vi "Load Fuzzy Controller.vi"(5 "File Path":path, 7 "Open-Dialog":string="Open...") -> (0 "Controller out":T1={"Parameters"={"antecedance"=[{"ling.var."="Fuzzy-IN II", "x-min"=-10.0, "x-max"=10.0, "setarray"=[{"linguistic term"="NB", "color"=16711680, "points"=[-1.0, -1.0, -0.09999999999999998, -0.050000000000000044]}, {"linguistic term"="NS", "color"=3342438, "points"=[-0.09999999999999998, -0.050000000000000044, -0.050000000000000044, 0.0]}, {"linguistic term"="ZE", "color"=16724991, "points"=[-0.050000000000000044, 0.0, 0.0, 0.050000000000000044]}, {"linguistic term"="PS", "color"=255, "points"=[0.0, 0.050000000000000044, 0.050000000000000044, 0.10000000000000009]}, {"linguistic term"="PB", "color"=26214, "points"=[0.050000000000000044, 0.10000000000000009, 1.0, 1.0]}]}], "consequence"=[{"ling.var."="Fuzzy-OUT II", "x-min"=-10.0, "x-max"=10.0, "setarray"=[{"linguistic term"="NV", "color"=16711680, "points"=[-1.0, -1.0, -1.0, -1.0]}, {"linguistic term"="NED", "color"=3342438, "points"=[-0.5, -0.5, -0.5, -0.5]}, {"linguistic term"="NU", "color"=16724991, "points"=[0.0, 0.0, 0.0, 0.0]}, {"linguistic term"="PED", "color"=255, "points"=[0.5, 0.5, 0.5, 0.5]}, {"linguistic term"="PV", "color"=26214, "points"=[1.0, 1.0, 1.0, 1.0]}]}], "conclusions"=[0, 1, 2, 3, 4], "degree-of-support"=[1.0, 1.0, 1.0, 1.0, 1.0], "defu"=[{"inference"=0, "defumethod"=2, "modification"=TRUE, "precision"=0, "no consequence"=0, "defaultvalue"=0.0}]}, "Description"={"Info"={"Path"=path "/Mac IIsi/Work IIsi/Carsten&Stefan/Controller/Behaelter_P2.fc", "Controller Name"="Behaelter_P2.fc", "Date"="02.07.1996", "Time"="10:49 Uhr"}, "Author"="", "Description"=""}} {"Parameters"."defu"."defaultvalue" format="%.2f"; "Parameters"."degree-of-support" step=0.009999999776482582 format="%.2f"; "Parameters"."consequence"."x-min" step=0.009999999776482582 format="%.2f"; "Parameters"."consequence"."x-max" step=0.009999999776482582 format="%.2f"; "Parameters"."consequence"."setarray"."points" step=0.009999999776482582 format="%.2f"; "Parameters"."antecedance"."x-min" step=0.009999999776482582 format="%.2f"; "Parameters"."antecedance"."x-max" step=0.009999999776482582 format="%.2f"; "Parameters"."antecedance"."setarray"."points" step=0.009999999776482582 format="%.2f"}, 1 "cancel":bool, 2 "error out":errorcluster, 3 "anteced. data range minimums":dbl[](array[numeric]) format="%.2f", 4 "anteced. data range maximums":dbl[](array[numeric]) format="%.2f", 6 "input name 1":string, 8 "min 1":dbl format="%.2f", 10 "input name 2":string, 11 "min 4":dbl format="%.2f", 12 "input name 4":string, 13 "min 3":dbl format="%.2f", 14 "input name 3":string, 15 "min 2":dbl format="%.2f")   [LabVIEW 2020, in "NI_fuzzy logic.lvlib"]
doc: "This VI loads all controller parameters and information. Use this VI together with Fuzzy Controller VI to implement a fuzzy controller designed with the Fuzzy Logic Controller Design project manager. The data file uses the .fc file extension."
uses:
  <vilib>/addons/control/fuzzy/NI_fuzzy logic.lvlib
  <vilib>/addons/control/fuzzy/fuzzy logic.llb/Fuzzy Datatype.ctl
panel:
  in  "error in (not an error)":errorcluster
  in  "Controller data":T2={"Parameters"={"antecedance"=[{"ling.var."="in1", "x-min"=-1.0, "x-max"=1.0, "setarray"=[{"linguistic term"="NE1", "color"=16711680, "points"=[-1.0, -1.0, -1.0, -2.2351741790771484e-05]}, {"linguistic term"="ZE1", "color"=255, "points"=[-1.0, 0.0, 0.0, 1.0]}, {"linguistic term"="PO1", "color"=26214, "points"=[0.0, 1.0, 1.0, 1.0]}]}, {"ling.var."="in2", "x-min"=-1.0, "x-max"=1.0, "setarray"=[{"linguistic term"="NE2", "color"=16711680, "points"=[-1.0, -1.0, -1.0, 0.0]}, {"linguistic term"="ZE2", "color"=255, "points"=[-1.0, 0.0, 0.0, 1.0]}, {"linguistic term"="PO2", "color"=26214, "points"=[0.0, 1.0, 1.0, 1.0]}]}], "consequence"=[{"ling.var."="out", "x-min"=-1.0, "x-max"=1.0, "setarray"=[{"linguistic term"="NEo", "color"=16711680, "points"=[-1.0, -1.0, -1.0, 0.0]}, {"linguistic term"="ZEo", "color"=255, "points"=[-1.0, 0.0, 0.0, 1.0]}, {"linguistic term"="POo", "color"=26214, "points"=[0.0, 1.0, 1.0, 1.0]}]}], "conclusions"=[3, 3, 3, 3, 3, 3, 3], "degree-of-support"=[1.0, 1.0, 1.0, 1.0, 1.0, 1.0, 1.0], "defu"=[{"inference"=0, "defumethod"=0, "modification"=TRUE, "precision"=0, "no consequence"=0, "defaultvalue"=0.0}]}, "Description"={"Info"={"Path"=path "/HD 1000/Desktop Folder/fuzzylab today/loadsave.vi", "Controller Name"="", "Date"="", "Time"=""}, "Author"="", "Text"=""}} {"Parameters"."defu"."defaultvalue" format="%.2f"; "Parameters"."degree-of-support" step=0.009999999776482582 format="%.2f"; "Parameters"."consequence"."x-min" step=0.009999999776482582 format="%.2f"; "Parameters"."consequence"."x-max" step=0.009999999776482582 format="%.2f"; "Parameters"."consequence"."setarray"."points" step=0.009999999776482582 format="%.2f"; "Parameters"."antecedance"."x-min" step=0.009999999776482582 format="%.2f"; "Parameters"."antecedance"."x-max" step=0.009999999776482582 format="%.2f"; "Parameters"."antecedance"."setarray"."points" step=0.009999999776482582 format="%.2f"}
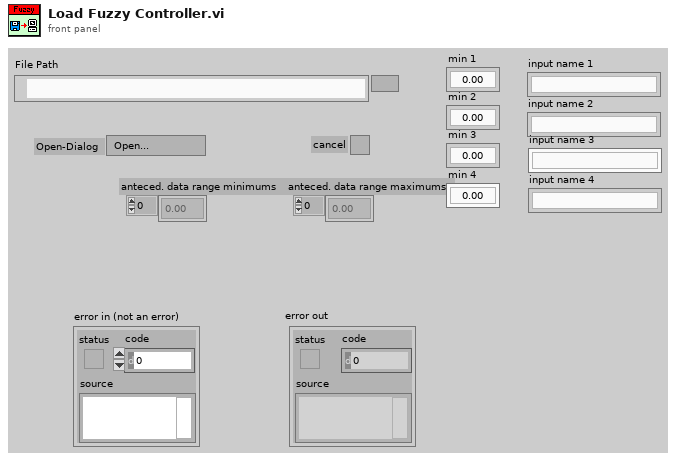
[diagram p1: front panel]
types:
  T1 = typedef "NI_fuzzy logic.lvlib/Fuzzy Datatype.ctl" = cluster{"Parameters":cluster{"antecedance":cluster{"ling.var.":string, "x-min":dbl, "x-max":dbl, "setarray":cluster{"linguistic term":string, "color":u32, "points":dbl[]}[]}[], "consequence":cluster{"ling.var.":string, "x-min":dbl, "x-max":dbl, "setarray":cluster{"linguistic term":string, "color":u32, "points":dbl[]}[]}[], "conclusions":u16[], "degree-of-support":dbl[], "defu":cluster{"inference":u16, "defumethod":u16, "modification":bool, "precision":u16, "no consequence":u16, "defaultvalue":dbl}[]}, "Description":cluster{"Info":cluster{"Path":path, "Controller Name":string, "Date":string, "Time":string}, "Author":string, "Description":string}}
  T2 = cluster{"Parameters":cluster{"antecedance":cluster{"ling.var.":string, "x-min":dbl, "x-max":dbl, "setarray":cluster{"linguistic term":string, "color":u32, "points":dbl[]}[]}[], "consequence":cluster{"ling.var.":string, "x-min":dbl, "x-max":dbl, "setarray":cluster{"linguistic term":string, "color":u32, "points":dbl[]}[]}[], "conclusions":u16[], "degree-of-support":dbl[], "defu":cluster{"inference":u16, "defumethod":u16, "modification":bool, "precision":u16, "no consequence":u16, "defaultvalue":dbl}[]}, "Description":cluster{"Info":cluster{"Path":path, "Controller Name":string, "Date":string, "Time":string}, "Author":string, "Text":string}}
  T3 = enum16{"open", "replace", "create", "open or create", "replace or create", "replace or create with confirmation"}
  T4 = cluster{"ling.var.":string, "x-min":dbl, "x-max":dbl, "setarray":cluster{"linguistic term":string, "color":u32, "points":dbl[]}[]}[]
  T5 = cluster{"inference":u16, "defumethod":u16, "modification":bool, "precision":u16, "no consequence":u16, "defaultvalue":dbl}[]
  T6 = cluster{"inference":u16, "defumethod":u16, "modification":bool, "precision":u16, "no consequence":u16, "defaultvalue":dbl}
  T7 = cluster{"linguistic term":string, "color":u32, "points":dbl[]}[]
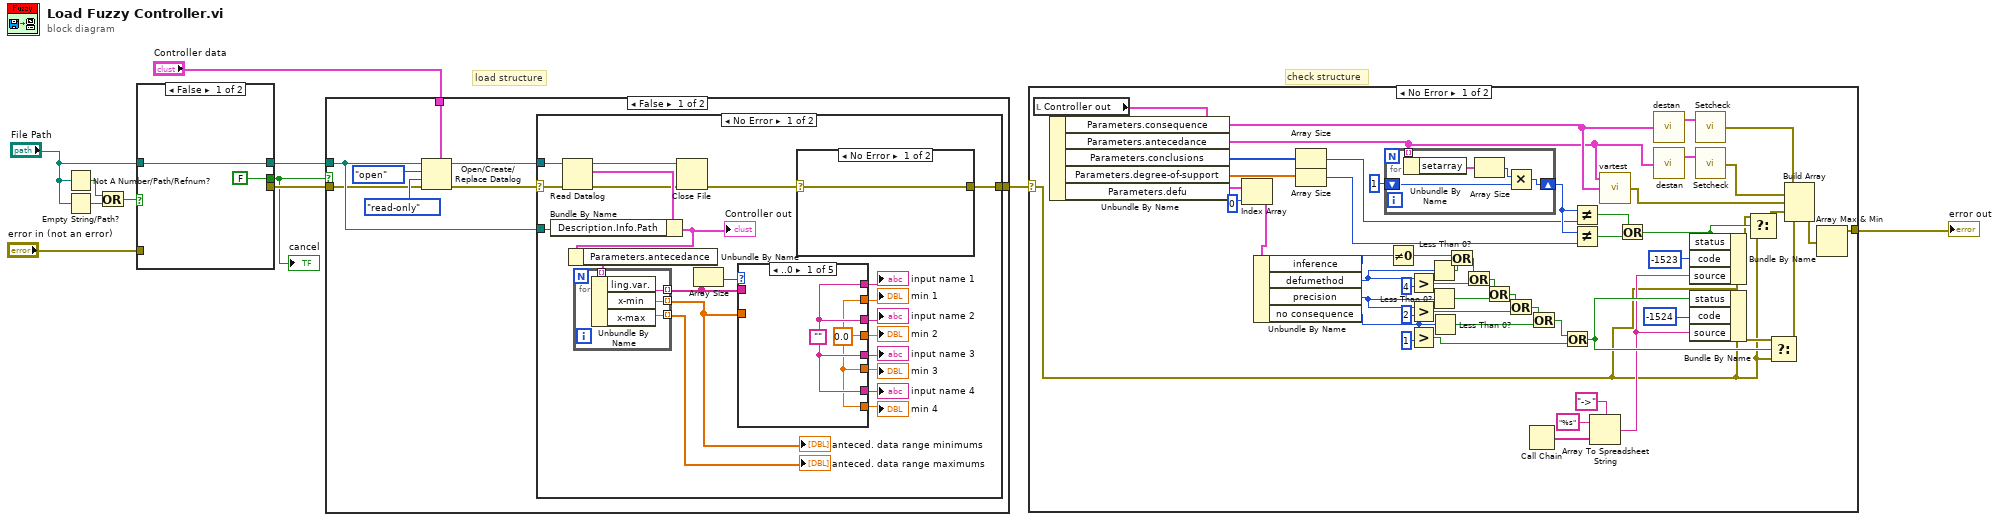
[diagram p0: block diagram]
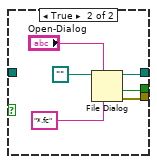
[diagram p2: hidden frame]
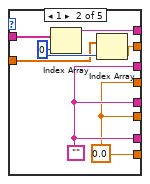
[diagram p4: hidden frame]
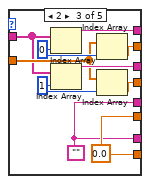
[diagram p5: hidden frame]
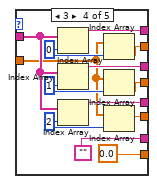
[diagram p6: hidden frame]
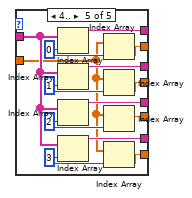
[diagram p7: hidden frame]
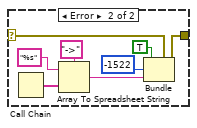
[diagram p8: hidden frame]
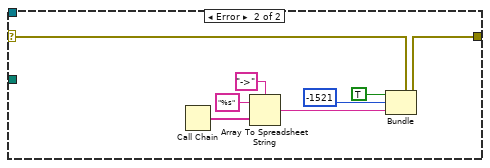
[diagram p9: hidden frame]
diagram:
  # "check structure"
  # "load structure"
  n1 = Not A Number/Path/Refnum?(number/path/refnum="File Path") -> (NaN/Path/Refnum?=w6:bool)
  n2 = Empty String/Path?(string/path="File Path") -> (empty?=w5:bool)
  n3 = Or(x=w6, y=w5) -> (x .or. y?=w3:bool)
  n4 = case shown="False" w3 {
    tunnel: [w13 w17] -> w9
    tunnel: [_ w19] -> w8
    tunnel: [FALSE ("cancelled") w18] -> w7
    tunnel: "File Path" -> [w13 _]
    tunnel: "error in (not an error)" -> [_ _]
    frame False {
    }
    frame True {
      n5 = File Dialog(6:"*.fc", 7:"Open-Dialog", 11:path "") -> (0:w19:errorcluster, 1:w18:bool, 3:w17:path)  [unwired: 1 in, 4 out]
    }
  }
  "cancel" <- w7
  n6 = case shown="False" w7 {
    tunnel: w9 -> [w25 _]
    tunnel: [w26 _] -> w1
    tunnel: "Controller data" -> [w24 _]
    tunnel: w8 -> [w21 _]
    frame False {
      n7 = Open/Create/Replace Datalog(5:w24, 8:w21, 9:enum16{"read/write", "read-only", "write-only"}."read-only" ("access (0:read/write)"), 10:T3."open" ("operation (0:open)"), 11:w25) -> (0:w20:errorcluster, 3:w27:refnum<k1>)  [unwired: 2 out]
      n8 = case shown="No Error" w20 {
        selector: w20 -> [w29 w113]
        tunnel: w27 -> [w49 _]
        tunnel: [w28 w109] -> w26
        tunnel: w25 -> [w46 _]
        frame No Error {
          n9 = Read Datalog(4:w29, 7:w49) -> (0:w31:errorcluster, 2:w47:T2, 3:w48:refnum<k1>)  [unwired: 1 out]
          n10 = Bundle By Name(cluster=w47, "Description.Info.Path"=w46) -> (w45:T2)
          "Controller out" <- w45
          n11 = Unbundle By Name(w45) -> ("Parameters.antecedance"=w44:T4)
          n12 = for {
            tunnel: w44 -> [w99] mode=indexing
            tunnel: [w98] -> w42 mode=indexing
            tunnel: [w97] -> w37 mode=indexing
            tunnel: [w96] -> w36 mode=indexing
            n13 = Unbundle By Name(w99) -> ("ling.var."=w98:string, "x-min"=w97:dbl, "x-max"=w96:dbl)
          }
          "anteced. data range minimums" <- w37
          "anteced. data range maximums" <- w36
          n14 = Close File(refnum=w48, error in=w31) -> (error out=w30:errorcluster)  [unwired: 1 out]
          n15 = Array Size(array=w42) -> (size(s)=w43:i32)
          n16 = case shown="..0" w43 {
            tunnel: w42 -> [_ w54 w60 w77 w90]
            tunnel: [w51 w58 w68 w81 w95] -> w41
            tunnel: [w51 w53 w66 w79 w93] -> w40
            tunnel: [w51 w53 w59 w78 w92] -> w39
            tunnel: [w51 w53 w59 "" w91] -> w38
            tunnel: w37 -> [_ w55 w62 w71 w82]
            tunnel: [w50 w56 w64 w74 w86] -> w35
            tunnel: [w50 w52 w63 w73 w85] -> w34
            tunnel: [w50 w52 w61 w72 w84] -> w33
            tunnel: [w50 w52 w61 0.0 w83] -> w32
            frame ..0 {
              w50 = 0.0
              w51 = ""
            }
            frame 1 {
              w52 = 0.0
              w53 = ""
              w57 = 0
              n17 = Index Array(array=w54, index=w57) -> (element=w58:string)
              n18 = Index Array(array=w55, index=w57) -> (element=w56:dbl)
            }
            frame 2 {
              w61 = 0.0
              w59 = ""
              w65 = 1
              w67 = 0
              n19 = Index Array(array=w60, index=w67) -> (element=w68:string)
              n20 = Index Array(array=w60, index=w65) -> (element=w66:string)
              n21 = Index Array(array=w62, index=w67) -> (element=w64:dbl)
              n22 = Index Array(array=w62, index=w65) -> (element=w63:dbl)
            }
            frame 3 {
              w75 = 2
              w76 = 1
              w80 = 0
              n23 = Index Array(array=w77, index=w80) -> (element=w81:string)
              n24 = Index Array(array=w77, index=w76) -> (element=w79:string)
              n25 = Index Array(array=w77, index=w75) -> (element=w78:string)
              n26 = Index Array(array=w71, index=w80) -> (element=w74:dbl)
              n27 = Index Array(array=w71, index=w76) -> (element=w73:dbl)
              n28 = Index Array(array=w71, index=w75) -> (element=w72:dbl)
            }
            frame 4.. {
              w87 = 3
              w88 = 2
              w89 = 1
              w94 = 0
              n29 = Index Array(array=w90, index=w94) -> (element=w95:string)
              n30 = Index Array(array=w90, index=w89) -> (element=w93:string)
              n31 = Index Array(array=w90, index=w88) -> (element=w92:string)
              n32 = Index Array(array=w90, index=w87) -> (element=w91:string)
              n33 = Index Array(array=w82, index=w94) -> (element=w86:dbl)
              n34 = Index Array(array=w82, index=w89) -> (element=w85:dbl)
              n35 = Index Array(array=w82, index=w88) -> (element=w84:dbl)
              n36 = Index Array(array=w82, index=w87) -> (element=w83:dbl)
            }
          }
          "input name 4" <- w38
          "input name 3" <- w39
          "input name 2" <- w40
          "input name 1" <- w41
          "min 4" <- w32
          "min 3" <- w33
          "min 2" <- w34
          "min 1" <- w35
          n37 = case shown="No Error" w30 {
            selector: w30 -> [w100 w103]
            tunnel: [w100 w101] -> w28
            frame No Error {
            }
            frame Error {
              n38 = Call Chain() -> (call chain=w106:string[])
              n39 = Array To Spreadsheet String(delimiter (Tab)="->", array=w106, 3:"%s" ("format string")) -> (spreadsheet string=w104:string)
              n40 = Bundle(cluster=w103, "status"=TRUE, "code"=-1522, "source"=w104) -> (w101:errorcluster)
            }
          }
        }
        frame Error {
          n41 = Call Chain() -> (call chain=w114:string[])
          n42 = Array To Spreadsheet String(delimiter (Tab)="->", array=w114, 3:"%s" ("format string")) -> (spreadsheet string=w110:string)
          n43 = Bundle(cluster=w113, "status"=TRUE, "code"=-1521, "source"=w110) -> (w109:errorcluster)
        }
      }
    }
    frame True {
      # "Operation Cancelled"
    }
  }
  n44 = case shown="No Error" w1 {
    selector: w1 -> [w117 w175]
    tunnel: [w159 w175] -> w11
    frame No Error {
      n45 = local read "Controller out"() -> (w169:T1)
      n46 = Unbundle By Name(w169) -> ("Parameters.consequence"=w128:T4, "Parameters.antecedance"=w125:T4, "Parameters.conclusions"=w167:u16[], "Parameters.degree-of-support"=w166:dbl[], "Parameters.defu"=w156:T5)
      n47 = Index Array(array=w156, index=0) -> (element=w154:T6)
      n48 = Unbundle By Name(w154) -> ("inference"=w153:u16, "defumethod"=w152:u16, "precision"=w148:u16, "no consequence"=w147:u16)
      n49 = Array Size(array=w167) -> (size(s)=w164:i32)
      n50 = Array Size(array=w166) -> (size(s)=w163:i32)
      n51 = for {
        tunnel: w125 -> [w174] mode=indexing
        shift-right: [w172] -> w165
        shift-left: 1 -> [w170]
        n52 = Unbundle By Name(w174) -> ("setarray"=w173:T7)
        n53 = Array Size(array=w173) -> (size(s)=w171:i32)
        n54 = Multiply(x=w171, y=w170) -> (x*y=w172:i32)
      }
      n55 = Not Equal To 0?(x=w153) -> (x != 0?=w146:bool)
      n56 = Greater?(x=w152, y=u16 4) -> (0:w143:bool)
      n57 = Greater?(x=w148, y=u16 2) -> (0:w139:bool)
      n58 = Greater?(x=w147, y=u16 1) -> (0:w135:bool)
      n59 = Less Than 0?(x=w152) -> (x < 0?=w145:bool)
      n60 = Less Than 0?(x=w148) -> (x < 0?=w141:bool)
      n61 = Less Than 0?(x=w147) -> (x < 0?=w137:bool)
      n62 = Or(x=w146, y=w145) -> (x .or. y?=w144:bool)
      n63 = Or(x=w144, y=w143) -> (x .or. y?=w142:bool)
      n64 = Or(x=w142, y=w141) -> (x .or. y?=w140:bool)
      n65 = Or(x=w140, y=w139) -> (x .or. y?=w138:bool)
      n66 = Call Chain() -> (call chain=w119:string[])
      n67 = Or(x=w138, y=w137) -> (x .or. y?=w136:bool)
      n68 = Or(x=w136, y=w135) -> (x .or. y?=w133:bool)
      n69 = Not Equal?(x=w165, y=w164) -> (x != y?=w162:bool)
      n70 = Not Equal?(x=w165, y=w163) -> (x != y?=w161:bool)
      n71 = Array To Spreadsheet String(delimiter (Tab)="->", array=w119, 3:"%s" ("format string")) -> (spreadsheet string=w118:string)
      n72 = call <vilib>:"vartest.vi"("consequencearray"=w128, "antecedancearray"=w125) -> ("error out"=w122:errorcluster)  [unwired: 1 out]
      n73 = Or(x=w162, y=w161) -> (x .or. y?=w160:bool)
      n74 = call <vilib>:"destan.vi"("variablearray"=w128) -> ("destandarized variable array"=w127:T4)
      n75 = call <vilib>:"destan.vi"("variablearray"=w125) -> ("destandarized variable array"=w126:T4)
      n76 = Bundle By Name(cluster=w117, "status"=w160, "code"=-1523, "source"=w118) -> (w132:errorcluster)
      n77 = Bundle By Name(cluster=w117, "status"=w133, "code"=-1524, "source"=w118) -> (w131:errorcluster)
      n78 = call <vilib>:"Setcheck.vi"("variablearray"=w127) -> ("error out"=w124:errorcluster)  [unwired: 1 in]
      n79 = call <vilib>:"Setcheck.vi"("variablearray"=w126) -> ("error out"=w123:errorcluster)  [unwired: 1 in]
      n80 = Select(t=w132, s=w160, f=w117) -> (s? t:f=w130:errorcluster)
      n81 = Select(t=w131, s=w133, f=w117) -> (s? t:f=w129:errorcluster)
      n82 = Build Array(w124, w123, w122, w130, w129) -> (w158:errorcluster[])
      n83 = Array Max & Min(array=w158) -> (max value=w159:errorcluster)  [unwired: 3 out]
    }
    frame Error {
      # "load-error in sequence 0"
    }
  }
  "error out" <- w11
